vi "getSlitPositionInMM.vi"(6 "Delay between send and receive [ms]":i32=100, 8 "error in (no error)":errorcluster, 10 "locationId":i32, 11 "Monochromator in":refnum<class "Monochromator.lvclass">) -> (0 "error out":errorcluster, 2 "position":dbl, 3 "Monochromator out":refnum<class "Monochromator.lvclass">)   [LabVIEW 2023, in "Monochromator.lvclass"]
uses:
  Monochromator.lvclass
  SlitPositionInMM.ctl
  de51f0bc-5a41-4012-b136-529a6c836e59.vi
  d9b87029-586e-44ee-a6e5-d4a5e0edce38.vi
  b59fd1e7-dcda-425c-bd6c-61aafb79e7f4.vi
  <vilib>/JDP Science/JSONtext/Variant to JSON Text.vi
  <vilib>/JDP Science/JSONtext/Set Item.vi
  <vilib>/JDP Science/JSONtext/JSON text to Variant.vi
  <vilib>/JDP Science/JSONtext/LVClass Serializer/JSONtext LVClass Serializer.lvclass
  Monochromator.lvclass/Monochromator.ctl
  GenericDevice/GenericDevice.lvclass
  <vilib>/IlluminatedG/lv-web-crypto/lv-json/JSON/JSON.lvlib
panel:
  # "Connector Pane"
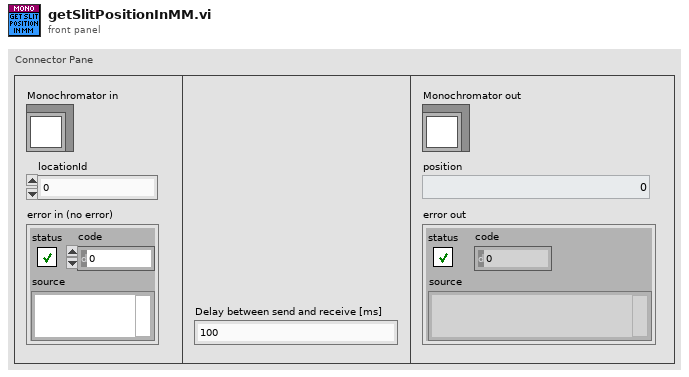
[diagram p1: front panel]
types:
  T1 = typedef "Monochromator.lvclass/SlitPositionInMM.ctl" = cluster{"locationId":dbl}
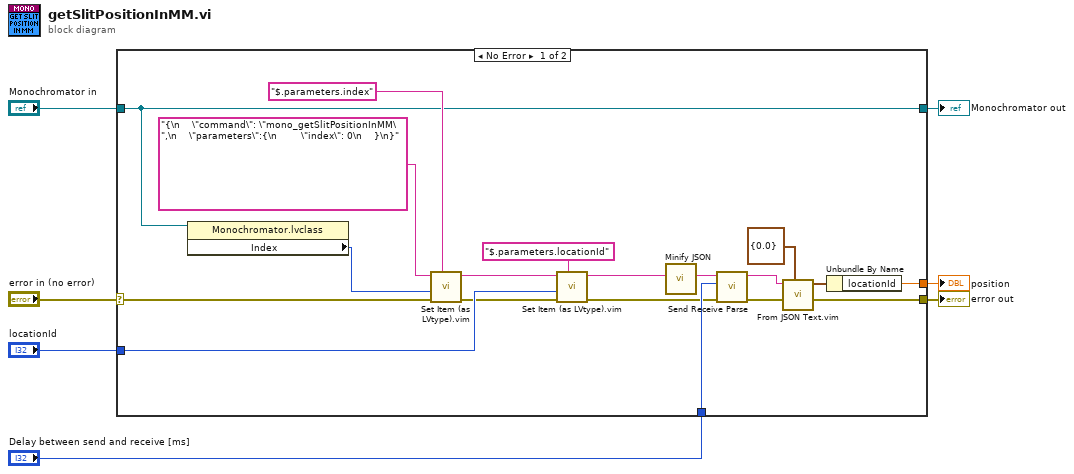
[diagram p0: block diagram]
diagram:
  n1 = case shown="No Error" "error in (no error)" {
    selector: "error in (no error)" -> [w14 w28]
    tunnel: [w25 w28] -> w6
    tunnel: [w16 w27] -> w4
    tunnel: "Monochromator in" -> [w16 w27]
    tunnel: "locationId" -> [w20 _]
    tunnel: [w11 _] -> w2
    tunnel: "Delay between send and receive [ms]" -> [w10 _]
    frame No Error {
      n2 = property class="Monochromator.lvclass"(reference=w16) -> ("Index"=w19:i32)  [unwired: 1 in, 2 out]
      n3 = call "Set Item (as LVtype).vim"("$Path or Item Name"="$.parameters.index", "error in (no error)"=w14, "Anything"=w19, "JSON"="{\n    \"command\": \"mono_getSlitPositionInMM\",\n    \"parameters\":{\n        \"index\": 0\n    }\n}") -> ("error out"=w13:errorcluster, "<JSON>"=w15:string)  [unwired: 4 in, 1 out]
      n4 = call "Set Item (as LVtype).vim"("$Path or Item Name"="$.parameters.locationId", "error in (no error)"=w13, "Anything"=w20, "JSON"=w15) -> ("error out"=w8:errorcluster, "<JSON>"=w9:string)  [unwired: 4 in, 1 out]
      n5 = call <vilib>:"Minify JSON.vi"("JSON String"=w9) -> ("Minified JSON"=w22:string)  [unwired: 10 in]
      n6 = call "Send Receive Parse.vi"("error in"=w8, "Delay between send and receive [ms]"=w10, "<JSON>"=w22) -> ("error out"=w23:errorcluster, "results-JSON string"=w24:string)  [unwired: 6 in, 1 out]
      n7 = call "From JSON Text.vim"("Data Type and Default Value"=T1 {"locationId"=0.0} ("slit position in mm"), "error in (no error)"=w23, "JSON"=w24) -> ("error out"=w25:errorcluster, "Data out"=w21:T1)  [unwired: 7 in]
      n8 = Unbundle By Name(w21) -> ("locationId"=w11:dbl)
    }
    frame Error {
    }
  }
  "error out" <- w6
  "Monochromator out" <- w4
  "position" <- w2
